vi "sub_data-valid_check.vi"(11 "gps receive parsing array":string[](array[string])) -> (1 "wgs84-1":cluster{dbl, dbl}={126.72082016226, 37.37012814476}, 2 "utm-1":cluster{dbl, dbl}={530126.7583503594, 175270.68061157822} {"?" format="%#.6f"; "?" format="%.6f"}, 3 "mode check":bool)   [LabVIEW 2019]
panel:
  out "index":i32
  out "경도":string="126.72082016226"
  out "위도":string="37.37012814476"
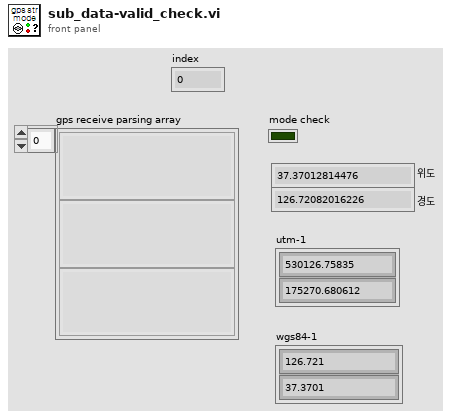
[diagram p1: front panel]
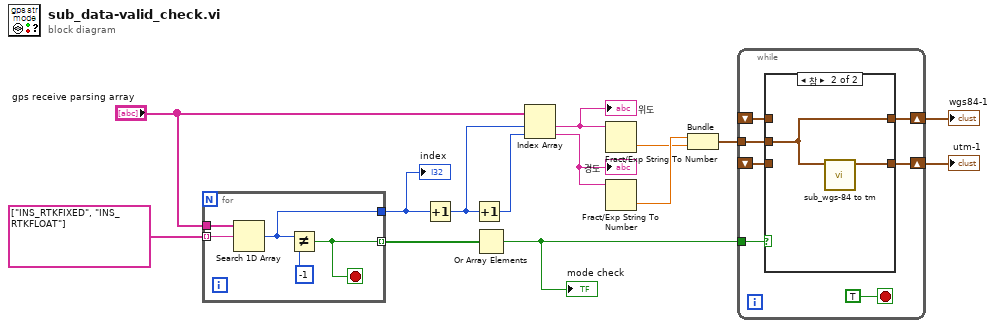
[diagram p0: block diagram]
diagram:
  n1 = for {
    tunnel: [w16] -> w14 mode=indexing
    tunnel: "gps receive parsing array" -> [w19]
    tunnel: string[] ["INS_RTKFIXED", "INS_RTKFLOAT"] -> [w17] mode=indexing
    tunnel: [w15] -> w4
    stop <- w16 stop-if-true
    n2 = Search 1D Array(1D array=w19, element=w17) -> (index of element=w15:i32)  [unwired: 1 in]
    n3 = Not Equal?(x=w15, y=-1) -> (x != y?=w16:bool)
  }
  "index" <- w4
  n4 = Increment(x=w4) -> (x+1=w8:i32)
  n5 = Increment(x=w8) -> (x+1=w7:i32)
  n6 = Or Array Elements(Boolean array=w14) -> (logical OR=w2:bool)
  "mode check" <- w2
  n7 = Index Array(array="gps receive parsing array", index #1=w8, index #2=w7) -> (element #1=w13:string, element #2=w12:string)
  "위도" <- w13
  "경도" <- w12
  n8 = Fract/Exp String To Number(string=w13) -> (number=w5:dbl)  [unwired: 3 in, 1 out]
  n9 = Fract/Exp String To Number(string=w12) -> (number=w6:dbl)  [unwired: 3 in, 1 out]
  n10 = Bundle(w6, w5) -> (w1:cluster{dbl, dbl})  [unwired: 1 in]
  n11 = while {
    tunnel: w2 -> [w25]
    shift-right: [w24] -> w9
    shift-left: _ -> [w22]
    shift-right: [w23] -> w10
    shift-left: _ -> [w21]
    tunnel: w1 -> [w20]
    stop <- TRUE stop-if-true
    n12 = case shown="참" w25 {
      tunnel: [w28 w29] -> w24
      tunnel: w20 -> [_ w29]
      tunnel: [w27 w30] -> w23
      tunnel: w22 -> [w28 _]
      tunnel: w21 -> [w27 _]
      frame False {
      }
      frame True {
        n13 = call "sub_wgs-84 to tm.vi"("in_lon-lat"=w29) -> ("TM"=w30:cluster{"Y(E)":dbl, "X(N)":dbl})  [unwired: 10 in]
      }
    }
  }
  "wgs84-1" <- w9
  "utm-1" <- w10
